vi "Init.vi"(10 "Node Data":T1, 11 "Node in":refnum<class "Node.lvclass">) -> (3 "Node out":refnum<class "Node.lvclass">)   [LabVIEW 2021, in "d20.lvlib" / "Node.lvclass"]
uses:
  Node.lvclass
  Node.lvclass/Node.ctl
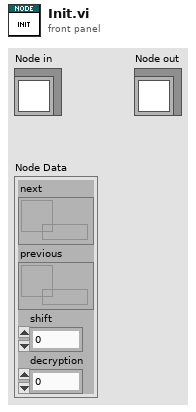
[diagram p1: front panel]
types:
  T1 = cluster{"next":refnum<data-value>, "previous":refnum<data-value>, "shift":i64, "decryption":i64}
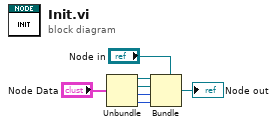
[diagram p0: block diagram]
diagram:
  n1 = Unbundle("Node Data") -> ("next"=w4:refnum<data-value>, "previous"=w3:refnum<data-value>, "shift"=w2:i64, "decryption"=w1:i64)
  n2 = Bundle(cluster="Node in", w4, w3, w2, w1) -> (→"Node out":refnum<class "Node.lvclass">)
